vi "Run Framework.vi"(5 "components directory":path, 7 "framework options":T13={"FIFO Options"={"Infinite Timeouts"=FALSE}, "Thread Options"={"Show FP On Call"=TRUE, "Close FP After Call"=TRUE, "Allow Debugging"=FALSE, "Restart On Error"=FALSE}, "Plugin Options"={"Default Components"=TRUE}, "Performance Options"={"Measure Period"=TRUE, "Measure Rx/Tx Duration"=TRUE}}, 8 "Actual Period":refnum<class "Pointer.lvclass">, 9 "Target Period":refnum<class "Pointer.lvclass">, 10 "Stop":refnum<class "Pointer.lvclass">, 11 "framework configuration":T1) -> ()   [LabVIEW 2017, in "DSF Core.lvlib"]
uses:
  DSF Core.lvlib
  Classes/Framework/Framework Options.ctl
  Typedefs/DSF FIFO Options.ctl
  Classes/Thread/DSF Thread Options.ctl
  Typedefs/DSF Plugin Options.ctl
  Typedefs/DSF Performance Options.ctl
  Typedefs/DSF Engine Framework Configuration.ctl
  Typedefs/DSF Engine Plugin Configuration.ctl
  Typedefs/DSF Timing Info.ctl
  Typedefs/DSF Engine Plugin Thread Configuration.ctl
  Typedefs/DSF Settings Info.ctl
  Typedefs/DSF Engine Transfer Group Configuration.ctl
  Typedefs/DSF Direction.ctl
  Typedefs/DSF Engine Transfer Configuration.ctl
  Typedefs/DSF Byte Order.ctl
  Typedefs/DSF Engine Channel Configuration.ctl
  Typedefs/DSF Data Type.ctl
  Typedefs/DSF Timeout Behavior.ctl
  <vilib>/NI/Memory Manager/Classes/Pointer/Pointer.lvclass
  <vilib>/NI/Memory Manager/Classes/Pointer/Pointer.lvclass/Pointer.ctl
  <vilib>/Platform/TimedLoop/XDataNode/timing_clust.ctl
  <vilib>/Platform/TimedLoop/XDataNode/nitl_modes.ctl
  <vilib>/Platform/TimedLoop/XDataNode/wakeup.ctl
  <vilib>/NI/Memory Manager/Classes/Pointer/Write U32.vi
  <vilib>/NI/Memory Manager/Classes/Pointer/Read U32.vi
  <vilib>/NI/Memory Manager/Classes/Pointer/Read Bool.vi
  <vilib>/NI/Memory Manager/Classes/Pointer/Write Bool.vi
  <vilib>/NI/Memory Manager/Classes/Pointer/Set Address.vi
  <vilib>/NI/Memory Manager/Classes/Pointer/Set Size.vi
  <vilib>/NI/Memory Manager/Classes/Pointer/Set Internal.vi
  <vilib>/NI/Memory Manager/Classes/Pointer/Check Null Pointer.vi
  <vilib>/NI/Memory Manager/Classes/Pointer/Clear (No Check).vi
  <vilib>/NI/Memory Manager/Classes/Pointer/Check Length.vi
  <vilib>/NI/Memory Manager/Classes/Pointer/Write (No Check).vi
  <vilib>/NI/Memory Manager/Classes/Pointer/Write (No Check) U32.vi
  <vilib>/NI/Memory Manager/Classes/Pointer/Check Move.vi
  <vilib>/NI/Memory Manager/Classes/Pointer/Read (No Check).vi
  <vilib>/NI/Memory Manager/Classes/Pointer/Read (No Check) U32.vi
  <vilib>/NI/Memory Manager/Classes/Pointer/Read (No Check) Bool.vi
  <vilib>/NI/Memory Manager/Classes/Pointer/Write (No Check) Bool.vi
  <vilib>/NI/Memory Manager/Classes/Pointer/Get Internal.vi
  <vilib>/NI/Memory Manager/Classes/Pointer/Errors.vi
  <vilib>/NI/Memory Manager/Classes/Pointer/Zone.vi
  <vilib>/NI/Memory Manager/Classes/Pointer/Null Pointer.vi
  <vilib>/NI/Memory Manager/Classes/Pointer/Is Null.vi
  <vilib>/NI/Memory Manager/Classes/Pointer/Check Bounds (Pointer).vi
  <vilib>/NI/Memory Manager/Classes/Pointer/Check Count.vi
  <vilib>/NI/Memory Manager/Classes/Pointer/Check Bounds (Power of 2).vi
  <vilib>/NI/Memory Manager/Classes/Pointer/Create Error.vi
  <vilib>/NI/Memory Manager/Classes/Pointer/Out of Bounds.vi
  <vilib>/NI/Memory Manager/Classes/Pointer/Check Bounds.vi
  <vilib>/NI/Memory Manager/Constants/Constants.vi
  <vilib>/NI/Memory Manager/Constants/Library Name.vi
  <vilib>/NI/Memory Manager/Classes/Pointer/Pointer Error Info.vi
  <vilib>/NI/Memory Manager/Constants/Pointer Class Name.vi
  <vilib>/NI/Memory Manager/Classes/Pointer/Write Pointer Size to Error.vi
  <vilib>/NI/Memory Manager/Classes/Pointer/Check Bounds (Buffer).vi
  <vilib>/NI/Memory Manager/Classes/Pointer/Buffer Underflow.vi
  <vilib>/NI/Memory Manager/VIs/New Error Cluster.vi
  <vilib>/NI/Memory Manager/VIs/New Error Cluster (512B).vi
  <vilib>/NI/Memory Manager/VIs/Set Error Status.vi
  <vilib>/NI/Memory Manager/VIs/Set Error Code.vi
  <vilib>/NI/Memory Manager/VIs/Set Error Source.vi
  <vilib>/NI/Memory Manager/VIs/Write String to Source.vi
  <vilib>/NI/Memory Manager/VIs/Write Numeric to Source.vi
  <vilib>/NI/Memory Manager/VIs/Write Numeric Scalar to Source (Base10 U64).vi
  Classes/Framework/Framework.lvclass
  <vilib>/platform/TimedLoop/XDataNode/XDataNode.xnode
  <vilib>/Platform/TimedLoop/XDataNode/XDNodeRunTimeDep.lvlib
panel:
  out "actual frequency":u32 format="%.0pHz"
  in  "target frequency":u32 format="%.0pHz"
  out "iteration":i32
  out "error out":errorcluster
  in  "stop":bool
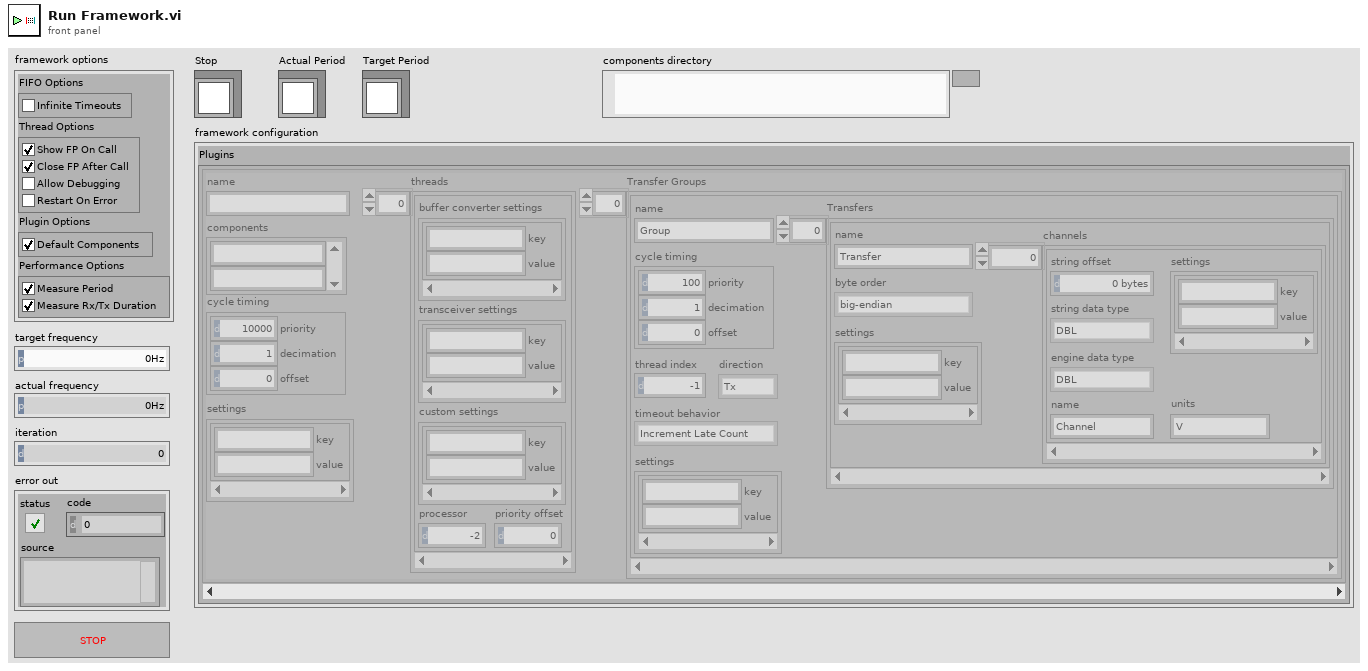
[diagram p1: front panel]
types:
  T1 = typedef "DSF Core.lvlib/DSF Engine Framework Configuration.ctl" = cluster{"Plugins":T2[]}
  T2 = typedef "DSF Core.lvlib/DSF Engine Plugin Configuration.ctl" = cluster{"name":string, "components":string[], "cycle timing":T3, "threads":T4[], "Transfer Groups":T6[], "settings":T5}
  T3 = typedef "DSF Core.lvlib/DSF Timing Info.ctl" = cluster{"priority":u64, "decimation":u64, "offset":u64}
  T4 = typedef "DSF Core.lvlib/DSF Engine Plugin Thread Configuration.ctl" = cluster{"buffer converter settings":T5, "transceiver settings":T5, "custom settings":T5, "processor":i32, "priority offset":i16}
  T5 = typedef "DSF Core.lvlib/DSF Settings Info.ctl" = cluster{"key":string, "value":string}[]
  T6 = typedef "DSF Core.lvlib/DSF Engine Transfer Group Configuration.ctl" = cluster{"name":string, "direction":T7, "cycle timing":T3, "thread index":i32, "settings":T5, "Transfers":T8[], "timeout behavior":T12}
  T7 = typedef "DSF Core.lvlib/DSF Direction.ctl" = enum8{"Tx", "Rx"}
  T8 = typedef "DSF Core.lvlib/DSF Engine Transfer Configuration.ctl" = cluster{"name":string, "byte order":T9, "settings":T5, "channels":T10[]}
  T9 = typedef "DSF Core.lvlib/DSF Byte Order.ctl" = enum8{"big-endian", "little-endian"}
  T10 = typedef "DSF Core.lvlib/DSF Engine Channel Configuration.ctl" = cluster{"string offset":u64, "string data type":T11, "engine data type":T11, "name":string, "settings":T5, "units":string}
  T11 = typedef "DSF Core.lvlib/DSF Data Type.ctl" = enum8{"Bool", "SGL", "DBL", "I8", "I16", "I32", "I64", "U8", "U16", "U32", "U64"}
  T12 = typedef "DSF Core.lvlib/DSF Timeout Behavior.ctl" = enum8{"Increment Late Count", "Throw Error"}
  T13 = typedef "DSF Core.lvlib/Framework.lvclass/Framework Options.ctl" = cluster{"FIFO Options":T14, "Thread Options":T15, "Plugin Options":T16, "Performance Options":T17}
  T14 = typedef "DSF Core.lvlib/DSF FIFO Options.ctl" = cluster{"Infinite Timeouts":bool}
  T15 = typedef "DSF Core.lvlib/DSF Thread Options.ctl" = cluster{"Show FP On Call":bool, "Close FP After Call":bool, "Allow Debugging":bool, "Restart On Error":bool}
  T16 = typedef "DSF Core.lvlib/DSF Plugin Options.ctl" = cluster{"Default Components":bool}
  T17 = typedef "DSF Core.lvlib/DSF Performance Options.ctl" = cluster{"Measure Period":bool, "Measure Rx/Tx Duration":bool}
  T18 = typedef "XDNodeRunTimeDep.lvlib/timing_clust.ctl" = cluster{"Expected End [f-1]":u64, "Actual End [f-1]":u64, "Finished Late? [f-1]":bool, "Expected End [i-1]":u64, "Actual End [i-1]":u64, "Finished Late? [i-1]":bool, "Expected Start [i]":u64, "Actual Start [i]":u64, "Expected Start [f]":u64, "Actual Start [f]":u64, "Source Name":string, "Structure Name":string, "Period":i64, "Deadline":i64, "Offset":i64, "Start":i64, "Priority":i32, "Timeout":i32, "Mode":T19, "Wakeup Reason":T20, "Error":errorcluster, "Source Type":string, "Secondary Source Type":string, "Global End Time":u64, "Global Start Time":u64, "Frame Duration":u64, "Iteration Duration":u64, "Assigned CPU":i32, "I/O Scan Engine Mode":u32}
  T19 = typedef "XDNodeRunTimeDep.lvlib/nitl_modes.ctl" = enum32{"No Change", "Process missed periods, maintain original phase", "Discard missed periods, maintain original phase", "Process missed periods, ignore original phase", "Discard missed periods, ignore original phase"}
  T20 = typedef "XDNodeRunTimeDep.lvlib/wakeup.ctl" = enum32{"Normal", "Aborted", "Asynchronous wakeup", "Timing source error", "Timed loop error", "Timeout"}
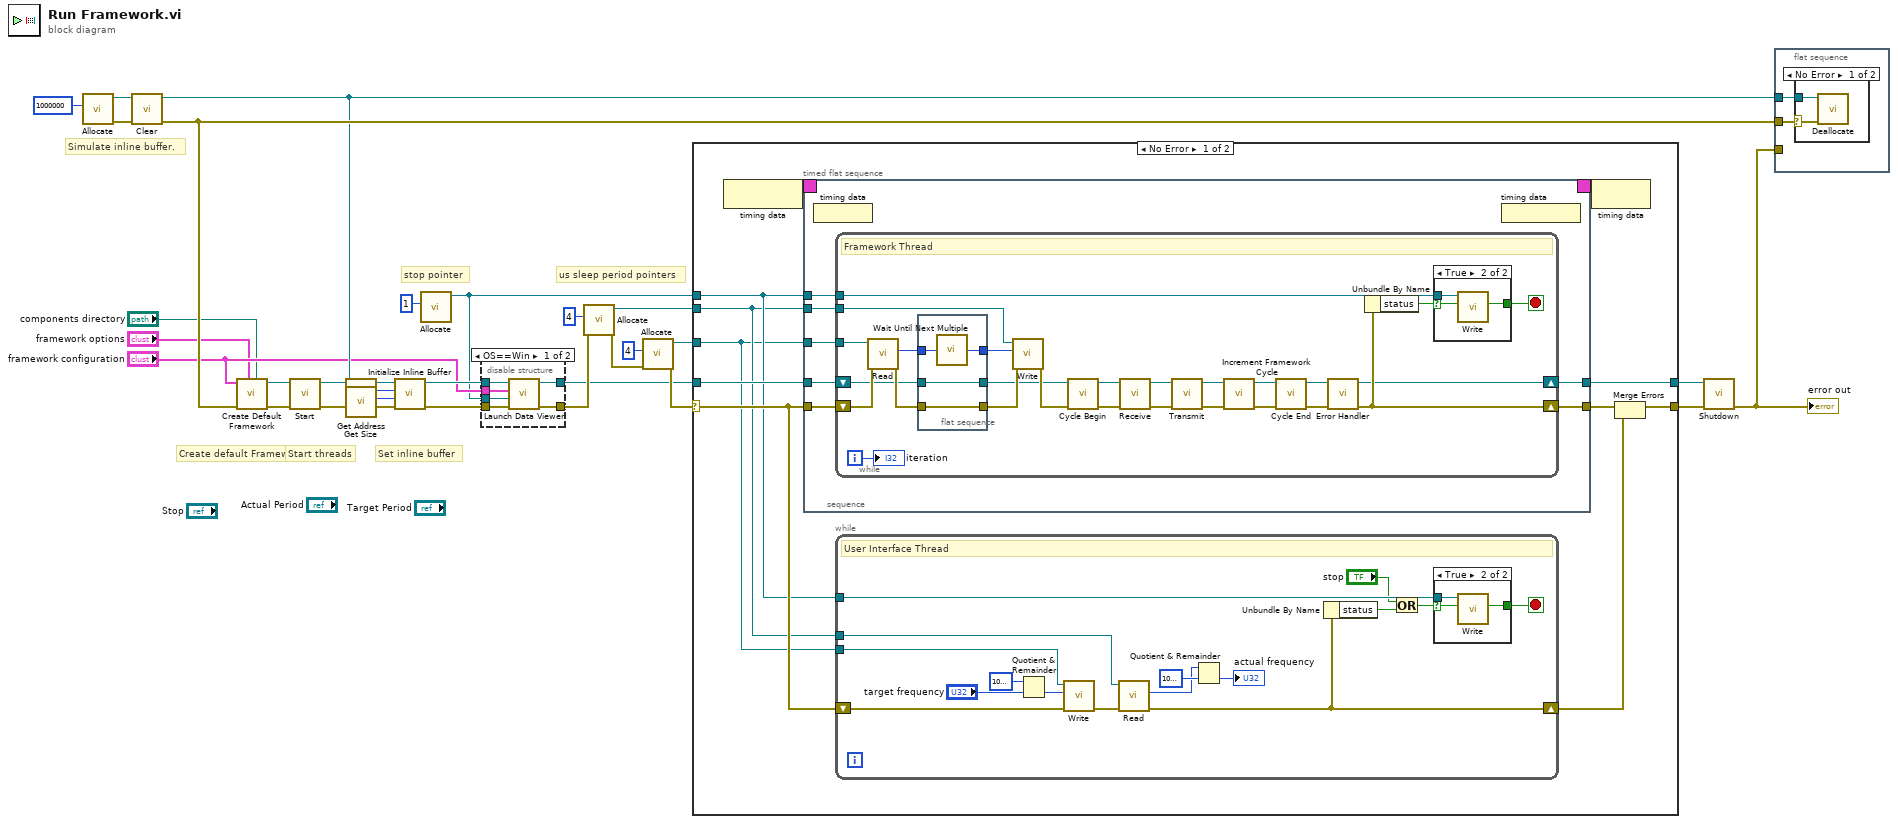
[diagram p0: block diagram]
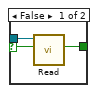
[diagram p4: hidden frame]
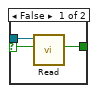
[diagram p5: hidden frame]
diagram:
  # "us sleep period pointers"
  # "stop pointer"
  # "Set inline buffer"
  # "Start threads"
  # "Create default Framework"
  # "Simulate inline buffer."
  n1 = call <vilib>:"Allocate.vi"("size"=u64 1000000) -> ("error out"=w24:errorcluster, "Pointer out"=w21:refnum<class "Pointer.lvclass">)  [unwired: 9 in]
  n2 = call <vilib>:"Clear.vi"("error in (no error)"=w24, "Pointer in"=w21) -> ("error out"=w29:errorcluster, "Pointer out"=w13:refnum<class "Pointer.lvclass">)  [unwired: 8 in]
  n3 = call "Create Default Framework.vi"("components directory (default)"="components directory", "framework options"="framework options", "error in (no error)"=w29, "framework configuration"="framework configuration") -> ("error out"=w15:errorcluster, "Framework"=w20:refnum<class "Framework.lvclass">)  [unwired: 6 in]
  n4 = call-dynamic "Start.vi"("error in (no error)"=w15, "Framework in"=w20) -> ("error out"=w19:errorcluster, "Framework out"=w28:refnum<class "Framework.lvclass">)  [unwired: 8 in]
  n5 = call <vilib>:"Get Address.vi"("Pointer in"=w13) -> ("address"=w22:u64)  [unwired: 9 in, 1 out]
  n6 = call <vilib>:"Get Size.vi"("Pointer in"=w13) -> ("size"=w23:u64)  [unwired: 9 in, 1 out]
  n7 = call "Initialize Inline Buffer.vi"("error in (no error)"=w19, "size"=w23, "address"=w22, "Framework in"=w28) -> ("error out"=w17:errorcluster, "Framework out"=w18:refnum<class "Framework.lvclass">)  [unwired: 6 in]
  n8 = call <vilib>:"Allocate.vi"("size"=u64 1) -> ("Pointer out"=w10:refnum<class "Pointer.lvclass">)  [unwired: 9 in, 1 out]
  n9 = disable-structure shown="OS==Win" {
    disable-tunnel: [w35 w37] -> w3
    disable-tunnel: [w34 w36] -> w4
    disable-tunnel: w18 -> [w33 w37]
    disable-tunnel: w17 -> [w32 w36]
    disable-tunnel: "framework configuration" -> [w31 _]
    disable-tunnel: w10 -> [w30 _]
    frame condition #0 (active) {
      n10 = call "Launch Data Viewer.vi"("error in (no error)"=w32, "Stop Pointer"=w30, "Framework Configuration"=w31, "Framework in"=w33) -> ("error out"=w34:errorcluster, "Framework out"=w35:refnum<class "Framework.lvclass">)  [unwired: 6 in]
    }
    frame condition #1 {
    }
  }
  n11 = call <vilib>:"Allocate.vi"("error in (no error)"=w4, "size"=u64 4) -> ("error out"=w5:errorcluster, "Pointer out"=w6:refnum<class "Pointer.lvclass">)  [unwired: 8 in]
  n12 = call <vilib>:"Allocate.vi"("error in (no error)"=w5, "size"=u64 4) -> ("error out"=w8:errorcluster, "Pointer out"=w9:refnum<class "Pointer.lvclass">)  [unwired: 8 in]
  n13 = case shown="No Error" w8 {
    selector: w8 -> [w48 w125]
    tunnel: [w39 w125] -> w27
    tunnel: w3 -> [w47 w126]
    tunnel: [w46 w126] -> w26
    tunnel: w10 -> [w43 _]
    tunnel: w9 -> [w41 _]
    tunnel: w6 -> [w42 _]
    frame No Error {
      n14 = node-c288() -> (w45:T18)
      n15 = timed-sequence {
        timing: w45 -> [_]
        timing-out: [_] -> w44
        tunnel: w47 -> [w77]
        tunnel: w48 -> [w76]
        tunnel: [w75] -> w46
        tunnel: [w74] -> w40
        tunnel: w43 -> [w73]
        tunnel: w41 -> [w72]
        tunnel: w42 -> [w71]
        n16 = timed-flat-sequence {
          tunnel: w77 -> [w84]
          tunnel: w76 -> [w83]
          tunnel: [w82] -> w75
          tunnel: [w81] -> w74
          tunnel: w73 -> [w80]
          tunnel: w72 -> [w79]
          tunnel: w71 -> [w78]
          n17 = node-c288() -> ()  [unwired: 1 in]
          n18 = while {
            shift-right: [w96] -> w82
            shift-left: w84 -> [w97]
            tunnel: w80 -> [w108]
            shift-right: [w102] -> w81
            shift-left: w83 -> [w99]
            tunnel: w79 -> [w100]
            tunnel: w78 -> [w91]
            i -> [w104]
            stop <- w107 stop-if-true
            # "Framework Thread"
            n19 = call-poly <vilib>:"Read.vi"("error in (no error)"=w99, "Pointer in"=w100) -> ("error out"=w98:errorcluster, "value out"=w101:u32)  [unwired: 6 in, 2 out]
            n20 = flat-sequence {
              tunnel: w97 -> [w114]
              tunnel: w98 -> [w113]
              tunnel: [w114] -> w92
              tunnel: [w113] -> w93
              tunnel: w101 -> [w112]
              tunnel: [w111] -> w95
              frame #0 {
                n21 = call "Wait Until Next Multiple"("Count(uSec)"=w112) -> ("Tick Count(uSec)"=w111:u32)
              }
            }
            n22 = call-poly <vilib>:"Write.vi"("error in (no error)"=w93, "value"=w95, "Pointer in"=w91) -> ("error out"=w94:errorcluster)  [unwired: 5 in, 3 out]
            n23 = call "Cycle Begin.vi"("error in (no error)"=w94, "Framework in"=w92) -> ("error out"=w105:errorcluster, "Framework out"=w106:refnum<class "Framework.lvclass">)  [unwired: 8 in]
            n24 = call "Receive.vi"("error in (no error)"=w105, "Framework in"=w106) -> ("error out"=w110:errorcluster, "Framework out"=w109:refnum<class "Framework.lvclass">)  [unwired: 8 in]
            n25 = call "Transmit.vi"("error in (no error)"=w110, "Framework in"=w109) -> ("error out"=w90:errorcluster, "Framework out"=w89:refnum<class "Framework.lvclass">)  [unwired: 8 in]
            n26 = call "Increment Framework Cycle.vi"("error in (no error)"=w90, "Framework in"=w89) -> ("error out"=w87:errorcluster, "Framework out"=w88:refnum<class "Framework.lvclass">)  [unwired: 8 in]
            n27 = call "Cycle End.vi"("error in (no error)"=w87, "Framework in"=w88) -> ("error out"=w86:errorcluster, "Framework out"=w85:refnum<class "Framework.lvclass">)  [unwired: 8 in]
            n28 = call "Error Handler.vi"("error in (no error)"=w86, "Framework in"=w85) -> ("error out"=w102:errorcluster, "Framework out"=w96:refnum<class "Framework.lvclass">)  [unwired: 8 in]
            n29 = Unbundle By Name(w102) -> ("status"=w103:bool)
            n30 = case shown="True" w103 {
              selector: w103 -> [w116 w119]
              tunnel: w108 -> [w117 w120]
              tunnel: [w115 w118] -> w107
              frame False {
                n31 = call-poly <vilib>:"Read.vi"("value in"=w116, "Pointer in"=w117) -> ("value out"=w115:bool)  [unwired: 6 in, 3 out]
              }
              frame True {
                n32 = call-poly <vilib>:"Write.vi"("value"=w119, "Pointer in"=w120) -> ("value"=w118:bool)  [unwired: 6 in, 3 out]
              }
            }
            "iteration" <- w104
          }
          n33 = node-c288() -> ()  [unwired: 1 out]
        }
      }
      n34 = while {
        tunnel: w43 -> [w64]
        shift-right: [w55] -> w38
        shift-left: w48 -> [w59]
        tunnel: w41 -> [w54]
        tunnel: w42 -> [w49]
        stop <- w63 stop-if-true
        # "User Interface Thread"
        n35 = Quotient & Remainder(x=u32 1000000 ("y"), y="target frequency") -> (floor(x/y)=w50:u32)  [unwired: 1 out]
        n36 = call-poly <vilib>:"Write.vi"("error in (no error)"=w59, "value"=w50, "Pointer in"=w54) -> ("error out"=w56:errorcluster)  [unwired: 5 in, 3 out]
        n37 = call-poly <vilib>:"Read.vi"("error in (no error)"=w56, "Pointer in"=w49) -> ("error out"=w55:errorcluster, "value out"=w51:u32)  [unwired: 6 in, 2 out]
        n38 = Quotient & Remainder(x=w51, y=u32 1000000) -> (floor(x/y)=→"actual frequency":u32)  [unwired: 1 out]
        n39 = Unbundle By Name(w55) -> ("status"=w61:bool)
        n40 = Or(x="stop", y=w61) -> (x .or. y?=w62:bool)
        n41 = case shown="True" w62 {
          selector: w62 -> [w66 w69]
          tunnel: w64 -> [w67 w70]
          tunnel: [w65 w68] -> w63
          frame False {
            n42 = call-poly <vilib>:"Read.vi"("value in"=w66, "Pointer in"=w67) -> ("value out"=w65:bool)  [unwired: 6 in, 3 out]
          }
          frame True {
            n43 = call-poly <vilib>:"Write.vi"("value"=w69, "Pointer in"=w70) -> ("value"=w68:bool)  [unwired: 6 in, 3 out]
          }
        }
      }
      n44 = node-c288(w44) -> ()
      n45 = Merge Errors(w40, w38) -> (w39:errorcluster)
    }
    frame Error {
    }
  }
  n46 = call-dynamic "Shutdown.vi"("error in (no error)"=w27, "Framework in"=w26) -> ("error out"=w14:errorcluster)  [unwired: 8 in, 1 out]
  "error out" <- w14
  n47 = flat-sequence {
    tunnel: w13 -> [w128]
    tunnel: w14 -> [_]
    tunnel: w29 -> [w127]
    frame #0 {
      n48 = case shown="No Error" w127 {
        selector: w127 -> [w129 _]
        tunnel: w128 -> [w130 _]
        frame No Error {
          n49 = call <vilib>:"Deallocate.vi"("error in (no error)"=w129, "Pointer"=w130) -> ()  [unwired: 8 in, 2 out]
        }
        frame Error {
        }
      }
    }
  }
